vi "grabber.vi"() -> ()   [LabVIEW 2010]
uses:
  scan_specification_tagResonant.ctl
  FPGA_ref.ctl
  <vilib>/Utility/error.llb/DialogType.ctl
  <vilib>/Platform/TimedLoop/XDataNode/XDataNode.xnode
  <vilib>/Platform/TimedLoop/XDataNode/timing_clust.ctl
  <vilib>/Platform/TimedLoop/XDataNode/nitl_modes.ctl
  <vilib>/Platform/TimedLoop/XDataNode/wakeup.ctl
  <vilib>/rvi/interface/nirviReadWriteControl/nirviReadWriteControl.xnode
  <vilib>/rvi/interface/common/niFpgaNodeNameForErrorReporting.ctl
  <vilib>/rvi/errors/niLvFpgaWhatHappensToTopLevelVI.ctl
  tracker status.ctl
  location3D.ctl
  <vilib>/dex/Flush And Wait Empty Condition.ctl
  <vilib>/rvi/interface/nirviMethod/nirviMethod.xnode
  <vilib>/rvi/interface/nirviCloseFPGA/nirviCloseFPGA.xnode
  common/utilities/get_time.vi
  sumLinesIntoVolume.vi
  addLineToVolume.vi
  get write location linear fit.vi
  <vilib>/Utility/error.llb/Error Cluster From Error Code.vi
  <vilib>/rvi/errors/niLvFpgaAdjustHostInterfaceError.vi
  <vilib>/FPGAPlugInAG/Dynamic/niLvFpga_Close_Dynamic.vi
  <vilib>/Platform/TimedLoop/XDataNode/XDNodeRunTimeDep.lvlib
  NiFpgaLv.dll
panel:
  in  "stim delay":i16=-10
  in  "BLEACH!":bool
  in  "Pockels cell bleach":i16=350 min=-750 max=750 step=1
  in  "pockels always on":bool
  in  "ff vel?":bool
  in  "lines per revolution":u16=50
  in  "mark valid location":bool
  in  "reset tracker":bool
  in  "number of spots":u8
  out "filtered spot locations":T1(array[cluster])
  in  "spot location constraints":T2(array[cluster])=[{"spot number"=0, "active"=FALSE, "x max"=0, "x min"=0, "y max"=0, "y min"=0}, {"spot number"=0, "active"=FALSE, "x max"=0, "x min"=0, "y max"=0, "y min"=0}, {"spot number"=0, "active"=FALSE, "x max"=0, "x min"=0, "y max"=0, "y min"=0}, {"spot number"=0, "active"=FALSE, "x max"=0, "x min"=0, "y max"=0, "y min"=0}]
  in  "inter-spot delay":u8
  in  "circles per spot":u16=4
  in  "stim width":u16=24 min=10
  out "stim laser on":bool
  in  "pos to stage lowpass f":dbl=20.0
  in  "measure offset":bool
  in  "Vxy feedback":bool=TRUE
  out "out of range":bool
  in  "auto disable tracking?":bool=TRUE
  in  "out of range (um)":dbl=220.0
  in  "pk-pk tag amplitude (um)":dbl=17.0
  in  "trackingToPiezoScale":fxp<+/-,16,5>=-0.43701171875
  out "current velocity":dbl[](array[numeric])
  out "current position":dbl[](array[numeric])
  in  "z-diff (um^2/ms)":dbl=1.0
  in  "Vz feedback?":bool
  in  "scale factors (um/level)":dbl[](array[numeric])=[0.016, 0.016, 0.00025]
  in  "z-feedback range":i16=5120
  in  "gaussian":bool=TRUE
  in  "x-y phase shift (*2^16/2*pi)":u16=16384
  in  "vmax (um/s)":dbl=10000.0
  in  "Vdiff /(g^2*1ms)":dbl=2e-08
  in  "r sphere/sigma (um)":dbl=3.0
  in  "min photons for update":u32=10
  in  "feedback channel":enum16{"channel 0", "channel 1", "both"}(ring)=enum."both"
  out "idle?":bool
  out "# elements in scan pos queue":i32
  in  "tracking?":bool
  in  "maximum galvo frequency":dbl=3000.0
  in  "scanning mode":enum16{"triangle", "spiral"}(ring)
  in  "LSB has acquire control":bool=TRUE
  in  "AI look-ahead":i16=1300
  in  "delay scan start":u16
  out "Queue Status":T3 {"lines that need sorting" format="%_3p"; "lines that need data" format="%.3p"}
  in  "xyz order":bool
  out "sorter stats":T4
  out "assembler status":T5
  in  "useReadPosition":bool=TRUE
  out "fpga update finished":bool
  out "transfer finished":bool
  out "assembler fin":bool
  out "finished":bool[](array[boolean])
  out "entered":bool[](array[boolean])
  in  "stop":bool
  in  "piezo z feedback":bool=TRUE
  in  "N Image sums":u32=20
  in  "spilt ff/fb":bool
  out "scan specification":T6={"z resolution (pixels)"=100, "iterations per pixel"=28, "iterations per z-scan (=zres*iterperpixel)"=50, "x resolution (pixels)"=100, "y resolution (pixels)"=80, "number of z-lines per volume"=30, "number of repetitions (volumes)"=5, "Pockels cell voltage (bits)"=80, "Vx center (bits)"=0, "Vy center (bits)"=0, "Vx amplitude (bits)"=40, "Vy amplitude (bits)"=0, "lines to delay between scan start and output"=1, "LSB has acquire control"=FALSE, "Pockels cell bleach voltage"=0}
  in  "Pockels cell voltage":i16=85 min=-750 max=750 step=1
  out "number of update commands received":i32
  out "scan spec set":bool
  out "display loop finished":bool
  in  "stop acquisition at FIFO overflow?":bool
  out "scanning? FPGA":bool
  in  "Close front-panel?":bool=TRUE
  out "initialised?":bool
  out "last received command":string
  out "command loop finished":bool
  out "read loop finished":bool
  out "scanning?":bool
  # "Status"
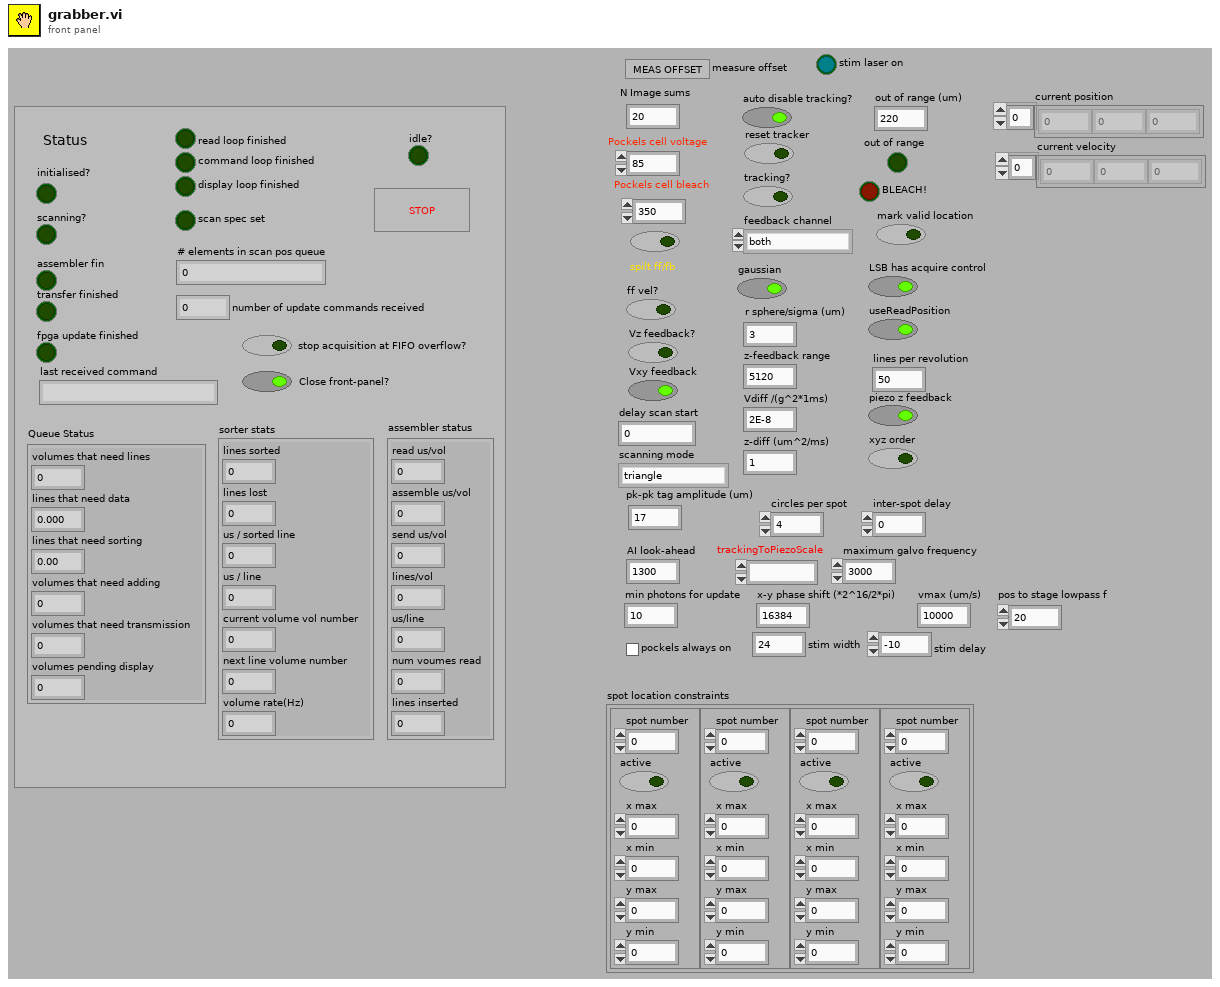
[diagram p1: front panel]
types:
  T1 = cluster{"Filtered x":dbl, "Filtered x":dbl, "Filtered x":dbl}[]
  T2 = cluster{"spot number":i8, "active":bool, "x max":i16, "x min":i16, "y max":i16, "y min":i16}[]
  T3 = cluster{"volumes that need lines":i32, "lines that need data":i32, "lines that need sorting":i32, "volumes that need adding":i32, "volumes that need transmission":i32, "volumes pending display":i32}
  T4 = cluster{"lines sorted":i32, "lines lost":i32, "us / sorted line":dbl, "us / line":dbl, "current volume vol number":u32, "next line volume number":u32, "volume rate(Hz)":dbl}
  T5 = cluster{"read us/vol":dbl, "assemble us/vol":dbl, "send us/vol":dbl, "lines/vol":dbl, "us/line":dbl, "num voumes read":u32, "lines inserted":i32}
  T6 = typedef "scan_specification_tagResonant.ctl" = cluster{"z resolution (pixels)":u16, "iterations per pixel":u16, "iterations per z-scan (=zres*iterperpixel)":u16, "x resolution (pixels)":u16, "y resolution (pixels)":u16, "number of z-lines per volume":u16, "number of repetitions (volumes)":i32, "Pockels cell voltage (bits)":i16, "Vx center (bits)":i16, "Vy center (bits)":i16, "Vx amplitude (bits)":i16, "Vy amplitude (bits)":i16, "lines to delay between scan start and output":u16, "LSB has acquire control":bool, "Pockels cell bleach voltage":i16}
  T7 = typedef "DialogType.ctl" = u16
  T8 = typedef "XDNodeRunTimeDep.lvlib/timing_clust.ctl" = cluster{"Expected End [f-1]":u64, "Actual End [f-1]":u64, "Finished Late? [f-1]":bool, "Expected End [i-1]":u64, "Actual End [i-1]":u64, "Finished Late? [i-1]":bool, "Expected Start [i]":u64, "Actual Start [i]":u64, "Expected Start [f]":u64, "Actual Start [f]":u64, "Source Name":string, "Structure Name":string, "Period":i64, "Deadline":i64, "Offset":i64, "Start":i64, "Priority":i32, "Timeout":i32, "Mode":T9, "Wakeup Reason":T10, "Error":errorcluster, "Source Type":string, "Secondary Source Type":string, "Global End Time":u64, "Global Start Time":u64, "Frame Duration":u64, "Iteration Duration":u64, "Assigned CPU":i32, "I/O Scan Engine Mode":u32}
  T9 = typedef "XDNodeRunTimeDep.lvlib/nitl_modes.ctl" = enum32{"No Change", "Process missed periods, maintain original phase", "Discard missed periods, maintain original phase", "Process missed periods, ignore original phase", "Discard missed periods, ignore original phase"}
  T10 = typedef "XDNodeRunTimeDep.lvlib/wakeup.ctl" = enum32{"Normal", "Aborted", "Asynchronous wakeup", "Timing source error", "Timed loop error", "Timeout"}
  T11 = typedef "internal_queues.ctl" = cluster{"volumeQueue":refnum<queue>, "linesWithoutDataQueue":refnum<queue>, "lineQueue":refnum<queue>, "volumesWithLinesQueue":refnum<queue>, "kalmanQueue":refnum<queue>, "completedVolumeQueue":refnum<queue>, "displayVolumeQueue":refnum<queue>, "scanLocationsQueue":refnum<queue>, "kalmanToDisplayPanel":refnum<queue>, "focalPositionQueue":refnum<queue>, "spotPositionsToImagePanel":refnum<queue>}
  T12 = typedef "network_streaming_queues_cluster.ctl" = cluster{"data writer endpoint":refnum<k21>, "command reader endpoint":refnum<k21>, "settings reader endpoint":refnum<k21>, "z/intensity tuples reader endpoint":refnum<k21>, "extra waitlines reader endpoint":refnum<k21>}
  T13 = typedef "FPGA_ref.ctl" = refnum<k20>
  T14 = cluster{"trackingPanel":refnum<vi>, "imagePanel":refnum<vi>, "fpgaDisplay":refnum<vi>, "stagePanel":refnum<vi>, "filePanel":refnum<vi>, "stimLaserPanel":refnum<vi>}
  T15 = typedef "niFpgaNodeNameForErrorReporting.ctl" = enum16{"Open FPGA VI Reference", "Read/Write Control", "Invoke Method: Abort", "Invoke Method: Acknowledge IRQ", "Invoke Method: Download", "Invoke Method: FIFO.Configure", "Invoke Method: FIFO.Read", "Invoke Method: FIFO.Start", "Invoke Method: FIFO.Stop", "Invoke Method: FIFO.Write", "Invoke Method: Reset", "Invoke Method: Run", "Invoke Method: Wait on IRQ", "Close FPGA VI Reference"}
  T16 = typedef "niLvFpgaWhatHappensToTopLevelVI.ctl" = enum16{"top level VI scripted behind XNode", "top level VI inlined behind XNode"}
  T17 = cluster{"scan specification":T6, "scale factors (um/level)":dbl[], "z-feedback range":i16, "r sphere/sigma (um)":dbl}
  T18 = cluster{"x min":i32, "x max":i32, "y min":i32, "y max":i32, "Active":bool}[]
  T19 = cluster{"x value":i16, "y value":i16, "z value":i16}[]
  T20 = cluster{"z resolution (pixels)":u16, "iterations per pixel":u16, "iterations per z-scan (=zres*iterperpixel)":u16, "x resolution (pixels)":u16, "y resolution (pixels)":u16, "number of z-lines per volume":u16, "number of repetitions (volumes)":i32, "Pockels cell voltage (bits)":i16, "Vx center (bits)":i16, "Vy center (bits)":i16, "Vx amplitude (bits)":i16, "Vy amplitude (bits)":i16, "lines to delay between scan start and output":u16, "LSB has acquire control":bool, "Pockels cell bleach voltage":i16}
  T21 = typedef "tracker status.ctl" = cluster{"scanning":bool, "tracking":bool, "out of range":bool, "stim laser on":bool}
  T22 = cluster{"None":i32, "Volume Start":i32, "Line Start":i32, "COM":i32, "not used":i32}
  T23 = cluster{"command elements pending":u32, "commands read":u32}
  T24 = typedef "location3D.ctl" = cluster{"x (um)":dbl, "y (um)":dbl, "z (um)":dbl, "time (ms)":i64}
  T25 = typedef "kalman_result_scaled.ctl" = cluster{"axis":u8, "pos":dbl, "vel":dbl, "wpe or z_piezo":dbl, "status":u32, "n photon ch 0":u32, "n photon ch 1":u32, "elapsed time":dbl}
  T26 = typedef "polar tracking settings.ctl" = cluster{"scan radius":u16, "2^16/lines per revolution":u16, "gx":fxp<+,16,8>, "rtw":fxp<+,16,26>, "lines per revolution":u8, "vel diff":fxp<+,24,-22>, "Dx - for pos only k-f":fxp<+,32,19>}
  T27 = cluster{"# elements in queue":i32, "# elements in queue":i32, "# elements in queue":i32, "# elements in queue":i32, "# elements in queue":i32, "# elements in queue":i32}
  T28 = typedef "Flush And Wait Empty Condition.ctl" = u8
  T29 = typedef "scan_specification_cluster.ctl" = cluster{"x amplitude":u16, "x resolution (pixels)":u16, "x offset fly-forward (iterations)":u16, "x offset fly-back (iterations)":u16, "y resolution (nr. of lines)":u16, "y step size":u16, "iterations per pixel":u16, "number of frames":i32, "y offset (pixels)":u16, "number of y-brake lines  (before y-fly-back)":u16, "number y-brake lines (after y-fly-back)":u16, "number of y-fly-back steps":u16, "lines per z step":u16, "number of z/intensity tuples":u16, "number of repetitions (volumes or planes)":i32, "z step size derived":u16, "choose the beginning of z scan":bool, "number of frames (settings)":i32, "FPGA trajectory?":bool, "Pockels cell voltage (bits)":i16, "Vy min(bits)":i16, "Vz min(bits)":i16}
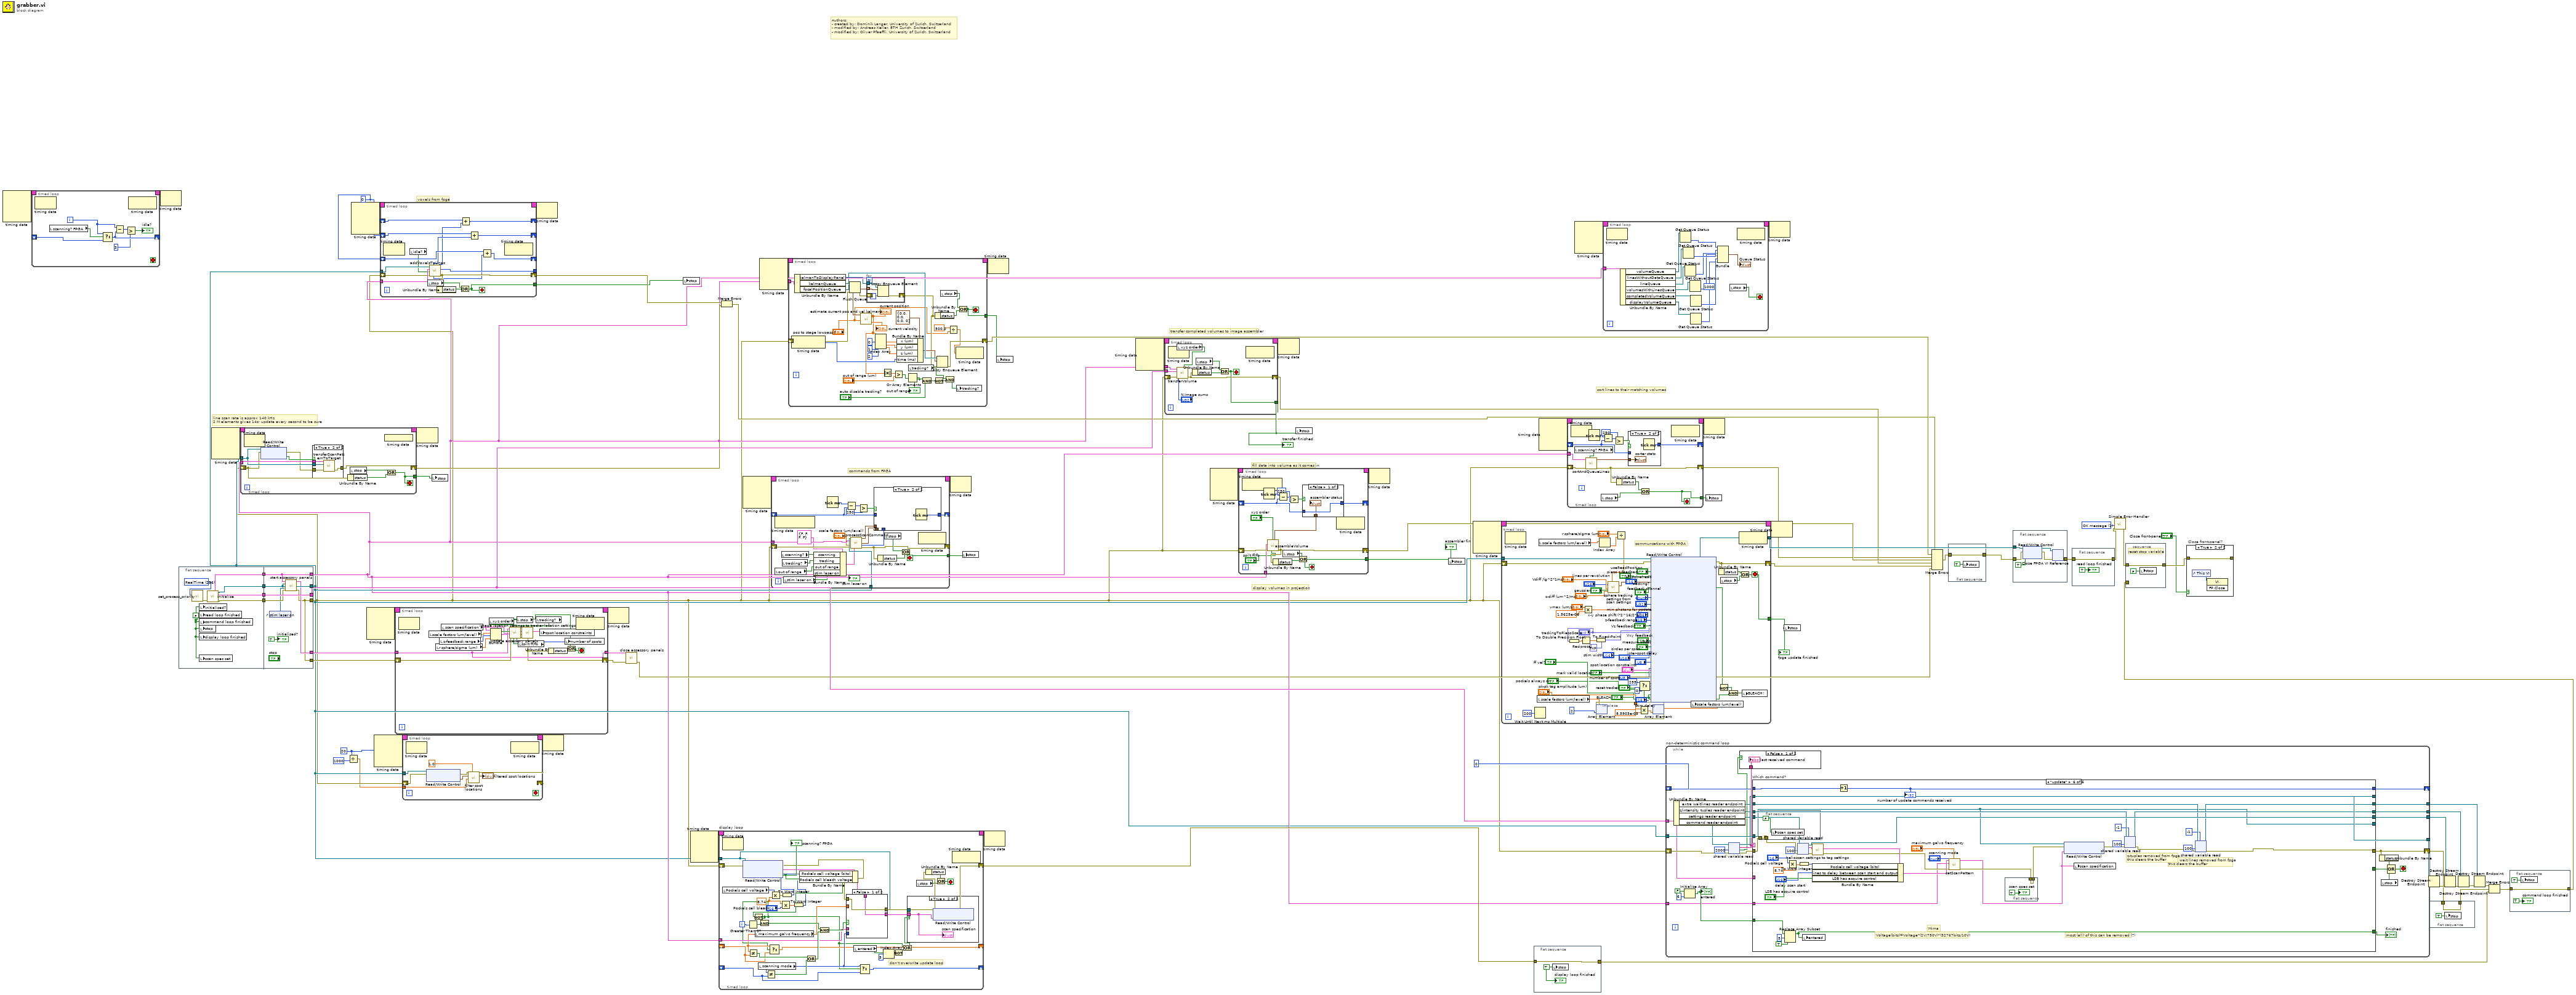
[diagram p0: block diagram]
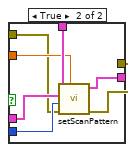
[diagram p3: hidden frame]
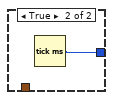
[diagram p6: hidden frame]
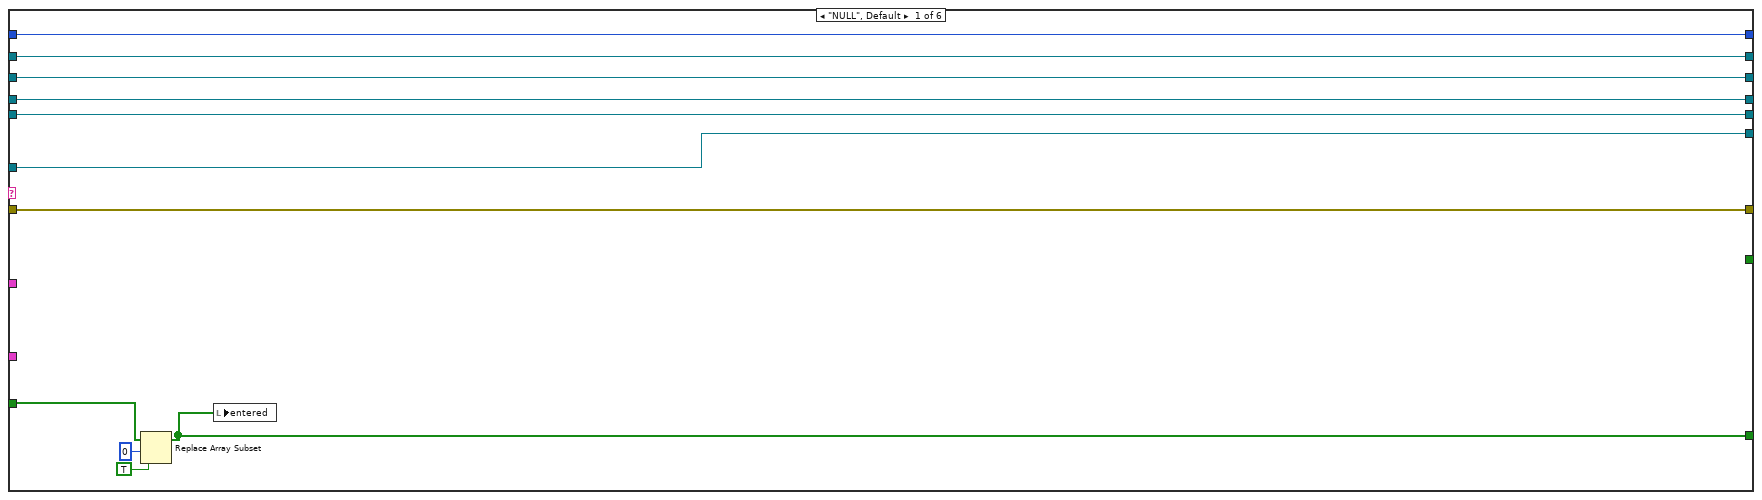
[diagram p10: hidden frame]
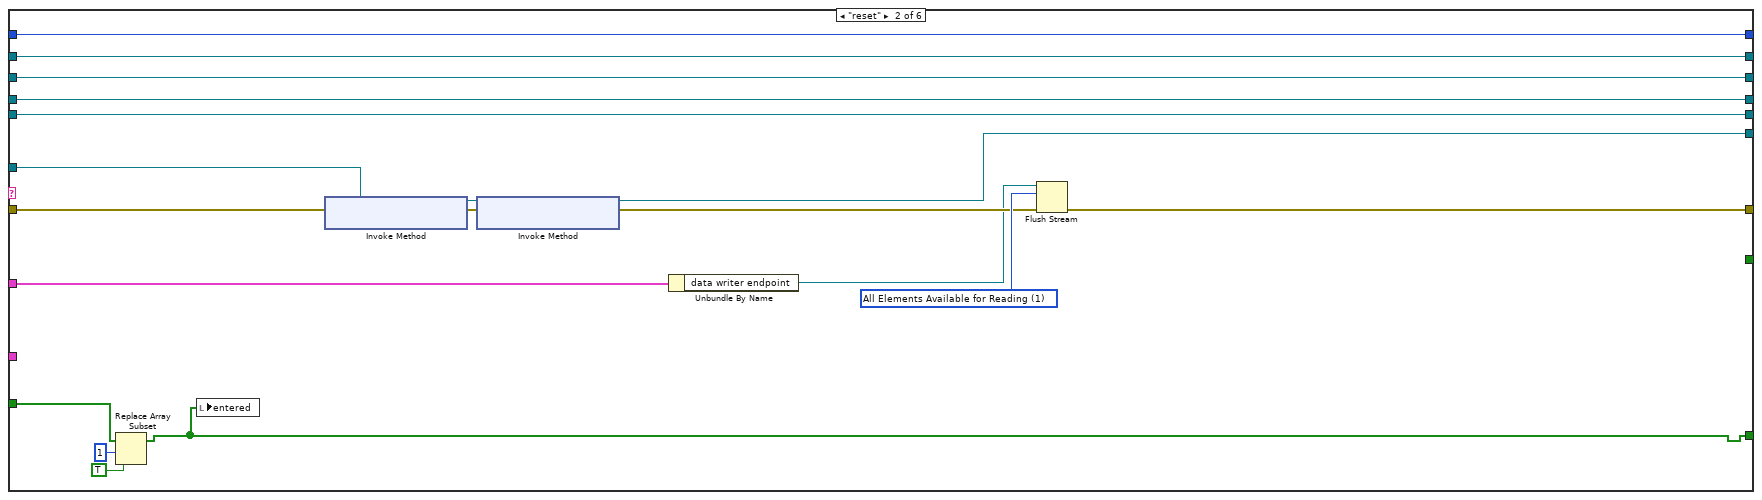
[diagram p11: hidden frame]
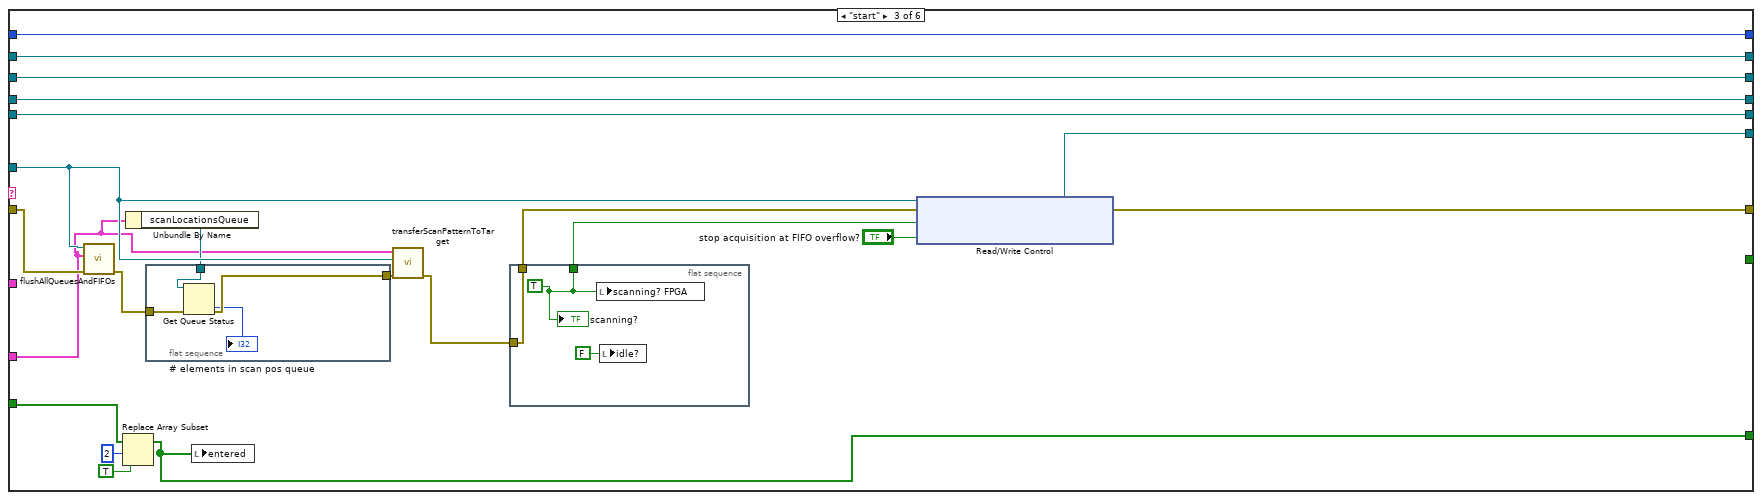
[diagram p12: hidden frame]
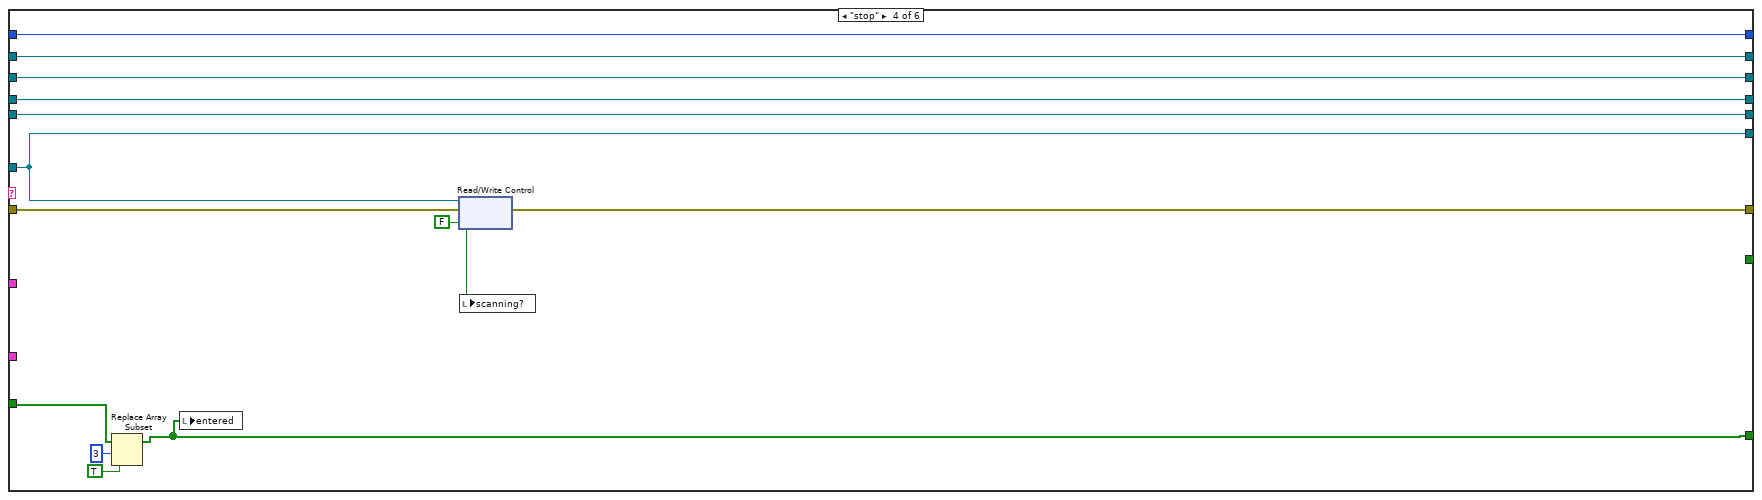
[diagram p13: hidden frame]
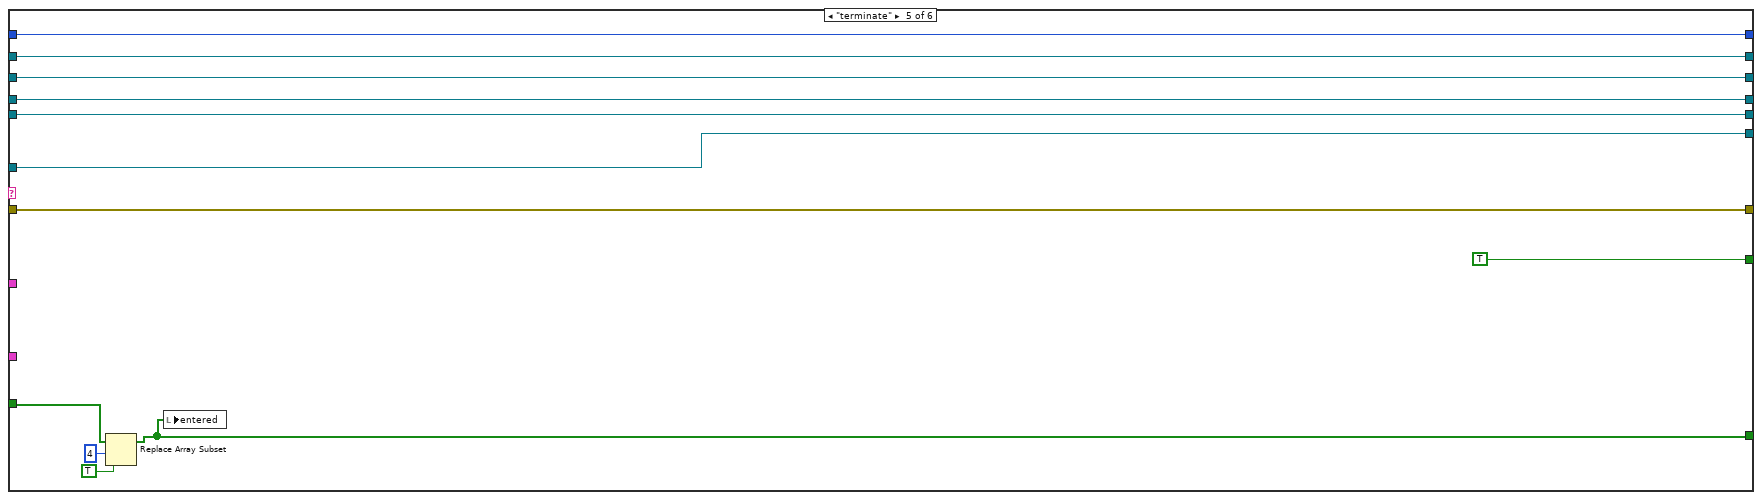
[diagram p14: hidden frame]
diagram:
  w3 = i64 20 ("Period")
  w27 = T7 1 items=["no dialog", "OK message", "continue or stop message", "OK message + warnings", "continue/stop + warnings"] ("type of dialog (OK msg:1)")
  w30 = u32 0
  # "sort lines to their matching volumes"
  # "line scan rate is approx 140 kHz\n2 M elements gives 14s; update every second to be sure"
  # "voxels from fpga"
  # "display volumes in projection"
  # "transfer completed volumes to image assembler"
  # "fill data into volume as it comes in"
  # "commands from FPGA"
  # "Authors: \n- created by: Dominik Langer, University of Zurich, Switzerland\n- modified by: Andreas Keller, ETH Zurich, Switzerland\n- modified by: Oliver Pfaeffli, University of Zurich, Switzerland"
  n1 = node-c288() -> (w23:T8)  [unwired: 4 in]
  n2 = timed-loop {
    timing: w23 -> [_]
    timing-out: [_] -> w22
    shift-right: [w88] -> _
    shift-left: _ -> [w90]
    i -> [w89]
    stop <- _ stop-if-true
    n3 = node-c288() -> ()  [unwired: 1 in, 1 out]
    n4 = local read "scanning? FPGA"() -> (w87:bool)
    n5 = Select(t=w89, s=w87, f=w90) -> (s? t:f=w88:i32)
    n6 = Subtract(x=w89, y=w88) -> (x-y=w86:i32)
    n7 = Greater?(x=w86, y=3) -> (0:→"idle?":bool)
    n8 = node-c288() -> ()  [unwired: 1 in, 1 out]
  }
  n9 = node-c288(w22) -> ()  [unwired: 1 out]
  n10 = flat-sequence {
    tunnel: [w97] -> w80
    tunnel: [w95] -> w79
    tunnel: [w96] -> w77
    tunnel: [w93] -> w61
    tunnel: [w104] -> w5
    tunnel: [w101] -> w4
    tunnel: w80 -> [w103]
    tunnel: w79 -> [w104]
    tunnel: [w106] -> w49
    tunnel: w77 -> [w106]
    tunnel: [w105] -> w31
    tunnel: w61 -> [w105]
    tunnel: [w102] -> w12
    tunnel: [w101] -> w11
    frame #0 {
      w94 = FALSE ("read loop finished")
      w99 = 256 items=["Normal"=32, "Idle"=64, "High"=128, "RealTime"=256, "BelowNormal"=16384, "AboveNormal"=32768] ("PriorityClass")
      n11 = call "set_process_priority.vi"("PriorityClass"=w99) -> ("error out"=w98:errorcluster)  [unwired: 10 in]
      n12 = local write "initialised?"(w94) -> ()
      n13 = local write "read loop finished"(w94) -> ()
      n14 = local write "command loop finished"(w94) -> ()
      n15 = local write "stop"(w94) -> ()
      n16 = local write "display loop finished"(w94) -> ()
      n17 = local write "scan spec set"(w94) -> ()
      n18 = call "initialise.vi"("error in (no error)"=w98) -> ("Queues"=w93:T11, "error out"=w97:errorcluster, "network streaming queues"=w96:T12, "FPGA VI ref"=w95:T13)  [unwired: 5 in, 1 out]
    }
    frame #1 {
      n19 = control-ref of="stim laser on"() -> (w100:refnum<vi>)
      n20 = call "start accessory panels.vi"("error in (no error)"=w103, "stim laser ref"=w100, "FPGA VI ref"=w104, "Queues"=w105) -> ("error out"=w101:errorcluster, "refs"=w102:T14)  [unwired: 6 in]
      "initialised?" <- TRUE ("initialised?")
    }
  }
  n21 = node-c288() -> (w46:T8)  [unwired: 4 in]
  n22 = timed-loop {
    shift-right: [w113] -> w35
    shift-left: w4 -> [w110]
    tunnel: w5 -> [w112]
    timing: w46 -> [_]
    timing-out: [_] -> w45
    tunnel: w31 -> [w114]
    tunnel: [w108] -> w25
    stop <- w108 stop-if-true
    n23 = node-c288() -> ()  [unwired: 1 in, 1 out]
    n24 = xnode "Read/Write Control"("FPGA VI Reference In"=w112, "error in"=w110) -> ("error out"=w109:errorcluster, "scanning?"=w111:bool)  [unwired: 1 out]
    n25 = case shown="True" w111 {
      tunnel: w109 -> [w117 w121]
      tunnel: w114 -> [_ w120]
      tunnel: [w117 w119] -> w113
      tunnel: w112 -> [_ w118]
      frame False {
      }
      frame True {
        n26 = call "transferScanPatternToTarget.vi"("error in (no error)"=w121, "FPGA VI ref"=w118, "Queues"=w120) -> ("error out"=w119:errorcluster)  [unwired: 8 in]
      }
    }
    n27 = Unbundle By Name(w110) -> ("status"=w116:bool)
    n28 = local read "stop"() -> (w115:bool)
    n29 = node-c288() -> ()  [unwired: 1 out]
    n30 = Or(x=w115, y=w116) -> (x .or. y?=w108:bool)
  }
  n31 = Divide(x=w3, y=i64 1000) -> (x/y=w1:dbl)
  n32 = node-c288() -> (w44:T8)  [unwired: 4 in]
  n33 = node-c288() -> (w14:T8)  [unwired: 4 in]
  n34 = node-c288(w3) -> (w7:T8)  [unwired: 3 in]
  n35 = timed-loop {
    timing: w44 -> [_]
    timing-out: [_] -> w43
    tunnel: w5 -> [w184]
    tunnel: w31 -> [w183]
    shift-right: [w178] -> w36
    shift-left: w4 -> [w180]
    tunnel: [w179] -> w26
    shift-right: [w177] -> _
    shift-left: w30 -> [w176]
    shift-right: [w175] -> _
    shift-left: w30 -> [w174]
    tunnel: [w173] -> _
    shift-right: [w169] -> _
    shift-left: w30 -> [w168]
    stop <- w179 stop-if-true
    n36 = node-c288() -> ()  [unwired: 1 in, 1 out]
    n37 = local read "idle?"() -> (w167:bool)
    n38 = local read "stop"() -> (w181:bool)
    n39 = call "addVoxelsToLines.vi"("error in"=w180, "idle?"=w167, "Queues"=w183, "FPGA VI ref"=w184) -> ("error out"=w178:errorcluster, "num elements available"=w173:u32, "num zero volume lines"=w170:u32, "num read"=w171:u32, "lines read"=w172:u32)  [unwired: 1 in, 2 out]
    n40 = Unbundle By Name(w178) -> ("status"=w182:bool)
    n41 = Or(x=w181, y=w182) -> (x .or. y?=w179:bool)
    n42 = Add(x=w168, y=w170) -> (x+y=w169:u32)
    n43 = Add(x=w176, y=w172) -> (x+y=w177:u32)
    n44 = Add(x=w174, y=w171) -> (x+y=w175:u32)
    n45 = node-c288() -> ()  [unwired: 1 in, 1 out]
  }
  n46 = timed-loop {
    timing: w14 -> [_]
    timing-out: [_] -> w13
    tunnel: w12 -> [w197]
    shift-right: [w192] -> w10
    shift-left: w11 -> [w200]
    tunnel: [w197] -> w9
    stop <- w198 stop-if-true
    n47 = node-c288() -> ()  [unwired: 1 in, 1 out]
    n48 = local read "scale factors (um/level)"() -> (w189:dbl[])
    n49 = local read "r sphere/sigma (um)"() -> (w187:dbl)
    n50 = local read "z-feedback range"() -> (w188:i16)
    n51 = local read "scan specification"() -> (w190:T6)
    n52 = local read "xyz order"() -> (w203:bool)
    n53 = Bundle("scan specification"=w190, "scale factors (um/level)"=w189, "z-feedback range"=w188, "r sphere/sigma (um)"=w187) -> (w191:T17)  [unwired: 1 in]
    n54 = local read "stop"() -> (w199:bool)
    n55 = local read "spilt ff/fb"() -> (w202:bool)
    n56 = local read "tracking?"() -> (w196:bool)
    n57 = call "update accessory panels.vi"("tracking"=w196, "spilt ff/fb"=w202, "xyz order"=w203, "error in (no error)"=w200, "scaling info"=w191, "stop"=w199, "refs"=w197) -> ("error out"=w192:errorcluster, "location constraints"=w194:T18, "num spots"=w195:u8)  [unwired: 2 in]
    n58 = call "image location settings to tracker location settings.vi"("scan settings"=w190, "location constraints"=w194) -> ("spot location constraints"=w193:T2)  [unwired: 9 in]
    n59 = local write "spot location constraints"(w193) -> ()
    n60 = Unbundle By Name(w192) -> ("status"=w201:bool)
    n61 = local write "number of spots"(w195) -> ()
    n62 = Or(x=w199, y=w201) -> (x .or. y?=w198:bool)
    n63 = node-c288() -> ()  [unwired: 1 in, 1 out]
  }
  n64 = timed-loop {
    timing: w7 -> [_]
    timing-out: [_] -> w6
    tunnel: w5 -> [w212]
    shift-right: [w209] -> _
    shift-left: w4 -> [w208]
    tunnel: w1 -> [w210]
    stop <- _ stop-if-true
    n65 = node-c288() -> ()  [unwired: 1 in, 1 out]
    n66 = xnode "Read/Write Control"("FPGA VI Reference In"=w212, "error in"=w208) -> ("error out"=w209:errorcluster, "Spot locations"=w211:T19)  [unwired: 1 out]
    n67 = call "filter spot locations.vi"("high cutoff freq: fh"=1.0, "sampling freq: fs"=w210, "Spot locations"=w211) -> ("filtered spot locations"=→"filtered spot locations":T1)  [unwired: 8 in]
    n68 = node-c288() -> ()  [unwired: 1 in, 1 out]
  }
  n69 = node-c288(w45) -> ()  [unwired: 1 out]
  n70 = local write "stop"(w25) -> ()
  n71 = node-c288(w43) -> ()  [unwired: 1 out]
  n72 = node-c288(w6) -> ()  [unwired: 1 out]
  n73 = node-c288(w13) -> ()  [unwired: 1 out]
  n74 = call "close accessory panels.vi"("error in (no error)"=w10, "refs"=w9) -> ("error out"=w8:errorcluster)  [unwired: 9 in]
  n75 = local write "stop"(w26) -> ()
  n76 = node-c288() -> (w17:T8)  [unwired: 4 in]
  n77 = timed-loop "display loop" {
    tunnel: w5 -> [w276]
    shift-right: [w288] -> w70
    shift-left: w4 -> [w302]
    shift-right: [w282] -> _
    shift-left: _ -> [w284]
    shift-right: [w285] -> _
    shift-left: _ -> [w287]
    tunnel: w31 -> [w290]
    timing: w17 -> [_]
    timing-out: [_] -> w16
    i -> [w298]
    stop <- w299 stop-if-true
    w268 = 8.74 ("x")
    # "don't overwrite update loop"
    n78 = node-c288() -> ()  [unwired: 1 in, 1 out]
    n79 = local read "Pockels cell voltage"() -> (w281:i16)
    n80 = xnode "Read/Write Control"("FPGA VI Reference In"=w276, "error in"=w302) -> ("error out"=w289:errorcluster, "scan specification"=w278:T20, "scanning?"=w296:bool)  [unwired: 1 out]
    "scanning? FPGA" <- w296
    n81 = Greater Than 0?(x=w298) -> (x > 0?=w297:bool)
    n82 = Not(x=w296) -> (.not. x?=w270:bool)
    n83 = local read "maximum galvo frequency"() -> (w283:dbl)
    n84 = Not Equal?(x=w283, y=w284) -> (x != y?=w294:bool)
    n85 = local read "scanning mode"() -> (w286:enum16{"triangle", "spiral"})
    n86 = And(x=w270, y=w297) -> (x .and. y?=w292:bool)
    n87 = Not Equal?(x=w286, y=w287) -> (x != y?=w295:bool)
    n88 = Select(t=w283, s=w270, f=w284) -> (s? t:f=w282:dbl)
    n89 = Multiply(x=w281, y=w268) -> (x*y=w280:dbl)
    n90 = Multiply(x=w268, y="Pockels cell bleach") -> (x*y=w266:dbl)
    n91 = To Word Integer(number=w280) -> (16bit integer=w279:i16)
    n92 = To Word Integer(number=w266) -> (16bit integer=w265:i16)
    n93 = Bundle By Name(cluster=w278, "Pockels cell voltage (bits)"=w279, "Pockels cell bleach voltage"=w265) -> (w277:T20)
    n94 = Or(x=w294, y=w295) -> (x .or. y?=w293:bool)
    n95 = And(x=w292, y=w293) -> (x .and. y?=w291:bool)
    n96 = case shown="False" w291 {
      tunnel: w277 -> [w351 w359]
      tunnel: w283 -> [_ w358]
      tunnel: w286 -> [_ w357]
      tunnel: w290 -> [_ w356]
      tunnel: [w352 w354] -> w288
      tunnel: w289 -> [w352 w355]
      tunnel: [w351 w353] -> w275
      frame False {
      }
      frame True {
        n97 = call "setScanPattern.vi"("maximum frequency"=w358, "error in (no error)"=w355, "scanning mode"=w357, "Queues"=w356, "scan specification - tag resonant"=w359) -> ("error out"=w354:errorcluster, "scan specification out"=w353:T6)  [unwired: 5 in]
      }
    }
    n98 = local read "entered"() -> (w274:bool[])
    n99 = Select(t=w286, s=w270, f=w287) -> (s? t:f=w285:enum16{"triangle", "spiral"})
    n100 = Index Array(array=w274, index=5) -> (element=w273:bool)
    n101 = Not(x=w273) -> (.not. x?=w271:bool)
    n102 = Or(x=w270, y=w271) -> (x .or. y?=w269:bool)
    n103 = case shown="True" w269 {
      tunnel: w276 -> [_ w304]
      tunnel: w275 -> [_ w303]
      frame False {
      }
      frame True {
        n104 = xnode "Read/Write Control"("FPGA VI Reference In"=w304, "scan specification"=w303) -> ()  [unwired: 1 in, 2 out]
        "scan specification" <- w303
      }
    }
    n105 = local read "stop"() -> (w300:bool)
    n106 = Unbundle By Name(w288) -> ("status"=w301:bool)
    n107 = Or(x=w301, y=w300) -> (x .or. y?=w299:bool)
    n108 = node-c288() -> ()  [unwired: 1 in, 1 out]
  }
  n109 = Merge Errors(w36, w35) -> (w34:errorcluster)
  n110 = node-c288() -> (w60:T8)  [unwired: 4 in]
  n111 = node-c288() -> (w21:T8)  [unwired: 4 in]
  n112 = timed-loop {
    tunnel: w5 -> [w458]
    shift-right: [w454] -> _
    shift-left: w4 -> [w455]
    timing: w60 -> [_]
    timing-out: [_] -> w59
    tunnel: w31 -> [w452]
    tunnel: [w453] -> w55
    shift-right: [w449] -> _
    shift-left: _ -> [w447]
    stop <- w453 stop-if-true
    n113 = node-c288() -> ()  [unwired: 1 in, 1 out]
    n114 = local read "out of range"() -> (w439:bool)
    n115 = local read "scanning?"() -> (w441:bool)
    n116 = local read "tracking?"() -> (w440:bool)
    n117 = local read "stim laser on"() -> (w438:bool)
    n118 = Bundle By Name(cluster=T21 {"scanning"=FALSE, "tracking"=FALSE, "out of range"=FALSE, "stim laser on"=FALSE} ("tracker status"), "scanning"=w441, "tracking"=w440, "out of range"=w439, "stim laser on"=w438) -> (w437:T21)
    n119 = Tick Count (ms)() -> (millisecond timer value=w448:u32)
    n120 = Subtract(x=w448, y=w447) -> (x-y=w446:u32)
    n121 = call "processScanCommand.vi"("FPGA VI Reference In"=w458, "Queues"=w452, "scale factors (um/level)"="scale factors (um/level)", "error in (no error)"=w455, "tracker status"=w437) -> ("num calls"=w451:T22, "command queue status"=w450:T23, "num kalmans per axis"=w436:u32[], "error out"=w454:errorcluster)  [unwired: 3 in, 4 out]
    n122 = Greater?(x=w446, y=u32 250) -> (0:w444:bool)
    n123 = case shown="True" w444 {
      tunnel: w451 -> [_ _]
      tunnel: w450 -> [_ _]
      tunnel: [w459 w460] -> w449
      tunnel: w447 -> [w459 _]
      tunnel: w436 -> [_ _]
      frame False {
      }
      frame True {
        n124 = Tick Count (ms)() -> (millisecond timer value=w460:u32)
      }
    }
    n125 = Unbundle By Name(w454) -> ("status"=w457:bool)
    n126 = local read "stop"() -> (w456:bool)
    n127 = Or(x=w456, y=w457) -> (x .or. y?=w453:bool)
    n128 = node-c288() -> ()  [unwired: 1 in, 1 out]
  }
  n129 = timed-loop {
    tunnel: w31 -> [w497]
    shift-right: [w476] -> w37
    shift-left: w4 -> [w495]
    timing: w21 -> [_]
    timing-out: [_] -> w20
    tunnel: [w488] -> w15
    stop <- w488 stop-if-true
    n130 = node-c288() -> (w480:i64)  [unwired: 1 in]
    n131 = Unbundle By Name(w497) -> ("kalmanToDisplayPanel"=w493:refnum<queue>, "kalmanQueue"=w496:refnum<queue>, "focalPositionQueue"=w479:refnum<queue>)
    n132 = Flush Queue(queue=w496, error in (no error)=w495) -> (remaining elements=w492:T25[], error out=w494:errorcluster)  [unwired: 1 out]
    n133 = call "estimate current pos and vel kalman.vi"("feedback lowpass f"="pos to stage lowpass f", "kalman updates"=w492) -> ("current velocity"=→"current velocity":dbl[], "current position"=w475:dbl[])  [unwired: 8 in]
    "current position" <- w475
    n134 = for {
      tunnel: w492 -> [w500] mode=indexing
      tunnel: w493 -> [w501]
      shift-right: [w498] -> w477
      shift-left: w494 -> [w499]
      n135 = Lossy Enqueue Element(queue=w501, element=w500, error in (no error)=w499) -> (error out=w498:errorcluster)  [unwired: 3 out]
    }
    n136 = Index Array(array=w475, index #1=0 ("index"), index #2=1 ("index"), index #3=2 ("index")) -> (element #1=w483:dbl, element #2=w482:dbl, element #3=w481:dbl)
    n137 = Absolute Value(x=w475) -> (abs(x)=w474:dbl[])
    n138 = Greater?(x=w474, y="out of range (um)") -> (0:w472:bool[])
    n139 = Bundle By Name(cluster=T24 {"x (um)"=0.0, "y (um)"=0.0, "z (um)"=0.0, "time (ms)"=0} ("location"), "x (um)"=w483, "y (um)"=w482, "z (um)"=w481, "time (ms)"=w480) -> (w478:T24)
    n140 = Or Array Elements(Boolean array=w472) -> (logical OR=w471:bool)
    "out of range" <- w471
    n141 = local read "tracking?"() -> (w467:bool)
    n142 = And(x=w471, y="auto disable tracking?") -> (x .and. y?=w469:bool)
    n143 = Not(x=w469) -> (.not. x?=w468:bool)
    n144 = Unbundle By Name(w477) -> ("status"=w490:bool)
    n145 = Lossy Enqueue Element(queue=w479, element=w478, error in (no error)=w477) -> (error out=w476:errorcluster)  [unwired: 3 out]
    n146 = local read "stop"() -> (w489:bool)
    n147 = And(x=w467, y=w468) -> (x .and. y?=w466:bool)
    n148 = Divide(x=500.0, y="pos to stage lowpass f") -> (x/y=w463:dbl)
    n149 = node-c288(w463) -> ()  [unwired: 1 out]
    n150 = local write "tracking?"(w466) -> ()
    n151 = Or(x=w489, y=w490) -> (x .or. y?=w488:bool)
  }
  n152 = node-c288(w59) -> ()  [unwired: 1 out]
  n153 = local write "stop"(w55) -> ()
  n154 = node-c288(w16) -> ()  [unwired: 1 out]
  n155 = node-c288(w20) -> ()  [unwired: 1 out]
  n156 = local write "stop"(w15) -> ()
  n157 = node-c288() -> (w40:T8)  [unwired: 4 in]
  n158 = timed-loop {
    tunnel: w31 -> [w508]
    shift-right: [w510] -> w48
    shift-left: w4 -> [w515]
    tunnel: [w512] -> w47
    tunnel: w49 -> [w509]
    timing: w40 -> [_]
    timing-out: [_] -> w39
    stop <- w512 stop-if-true
    n159 = node-c288() -> ()  [unwired: 1 in, 1 out]
    n160 = local read "xyz order"() -> (w507:bool)
    n161 = call "transferVolume.vi"("xyz order"=w507, "error in (no error)"=w515, "num vol to sum"="N Image sums", "network streaming queues"=w509, "Queues"=w508) -> ("error out"=w510:errorcluster)  [unwired: 1 in, 5 out]
    n162 = Unbundle By Name(w510) -> ("status"=w514:bool)
    n163 = local read "stop"() -> (w513:bool)
    n164 = Or(x=w513, y=w514) -> (x .or. y?=w512:bool)
    n165 = node-c288() -> ()  [unwired: 1 in, 1 out]
  }
  "transfer finished" <- w47
  n166 = node-c288() -> (w58:T8)  [unwired: 4 in]
  n167 = timed-loop {
    timing: w58 -> [_]
    timing-out: [_] -> w57
    tunnel: w31 -> [w527]
    shift-right: [w528] -> w53
    shift-left: w4 -> [w532]
    tunnel: [w529] -> w56
    shift-right: [w526] -> _
    shift-left: _ -> [w521]
    stop <- w529 stop-if-true
    n168 = node-c288() -> ()  [unwired: 1 in, 1 out]
    n169 = Tick Count (ms)() -> (millisecond timer value=w525:u32)
    n170 = call "assembleVolume.vi"("calc ff/fb"="spilt ff/fb", "error in (no error)"=w532, "xyz order"="xyz order", "Queues"=w527) -> ("error out"=w528:errorcluster, "status"=w520:T5)  [unwired: 5 in, 1 out]
    n171 = Unbundle By Name(w528) -> ("status"=w531:bool)
    n172 = Subtract(x=w525, y=w521) -> (x-y=w524:u32)
    n173 = local read "stop"() -> (w530:bool)
    n174 = Greater?(x=w524, y=u32 250) -> (0:w522:bool)
    n175 = Or(x=w530, y=w531) -> (x .or. y?=w529:bool)
    n176 = case shown="False" w522 {
      tunnel: [w534 w535] -> w526
      tunnel: w521 -> [w534 _]
      tunnel: w520 -> [w533 _]
      frame False {
        "assembler status" <- w533
      }
      frame True {
        n177 = Tick Count (ms)() -> (millisecond timer value=w535:u32)
      }
    }
    n178 = node-c288() -> ()  [unwired: 1 in, 1 out]
  }
  "assembler fin" <- w56
  n179 = node-c288(w39) -> ()  [unwired: 1 out]
  n180 = local write "stop"(w47) -> ()
  n181 = node-c288(w57) -> ()  [unwired: 1 out]
  n182 = local write "stop"(w56) -> ()
  n183 = node-c288() -> (w19:T8)  [unwired: 4 in]
  n184 = timed-loop {
    tunnel: w5 -> [w592]
    shift-right: [w555] -> w54
    shift-left: w4 -> [w591]
    tunnel: [w587] -> w51
    tunnel: [w586] -> w50
    timing: w19 -> [_]
    timing-out: [_] -> w18
    stop <- w586 stop-if-true
    # "communcations with FPGA"
    n185 = node-c288() -> ()  [unwired: 1 in, 1 out]
    n186 = Wait Until Next ms Multiple(millisecond multiple=u32 200) -> ()  [unwired: 1 out]
    n187 = local read "scale factors (um/level)"() -> (w566:dbl[])
    n188 = local read "scale factors (um/level)"() -> (w559:dbl[])
    n189 = To Double Precision Float(number="trackingToPiezoScale") -> (double precision float=w570:dbl)
    n190 = Reciprocal(x=w570) -> (1/x=w569:dbl)
    n191 = Multiply(x="vmax (um/s)", y=1.5625e-06) -> (x*y=w577:dbl)
    n192 = To Fixed-Point(fixed-point type=fxp<+/-,16,2> 0.0 ("piezoToTrackingScale"), number=w569) -> (fixed-point=w568:fxp<+/-,16,2>)
    n193 = in-place {
      in-place-border: "pk-pk tag amplitude (um)" -> [w596]
      n194 = in-place-array #1(w566, 2) -> ()  [unwired: 1 out]
      n195 = Multiply(x=w596, y=8.5903e-05) -> (x*y=w594:dbl)
      n196 = in-place-array #1(w594) -> (w565:dbl[])  [unwired: 1 out]
    }
    n197 = Index Array(array=w559) -> (element=w558:dbl)  [unwired: 1 in]
    n198 = Divide(x="r sphere/sigma (um)", y=w558) -> (x/y=w561:dbl)
    n199 = call "sphere tracking settings from scan settings.vi"("gaussian"="gaussian", "sphere radius/sigma"=w561, "z-diff (um^2/ms)"="z-diff (um^2/ms)", "Vdiff /(g^2*1ms)"="Vdiff /(g^2*1ms)", "lines per revolution"="lines per revolution") -> ("tracking settings out"=w581:T26)  [unwired: 6 in]
    n200 = Select(t=u8 255, s="reset tracker", f=u8 0) -> (s? t:f=w549:u8)
    n201 = xnode "Read/Write Control"("FPGA VI Reference In"=w592, "error in"=w591, "piezo z feedback"="piezo z feedback", "useReadPosition"="useReadPosition", "AI look-ahead"="AI look-ahead", "tracking settings"=w581, "tracking?"="tracking?", "feedback channel"="feedback channel", "min photons for update"="min photons for update", "vmax"=w577, "x-y phase shift (*2^16/2*pi)"="x-y phase shift (*2^16/2*pi)", "half valid z-range (ncycles * 64)"="z-feedback range", "Vz feedback?"="Vz feedback?", "trackingToPiezoScale"="trackingToPiezoScale", "piezoToTrackingScale"=w568, "Vxy feedback"="Vxy feedback", "measure offset"="measure offset", "stim buffer counts"="stim width", "circles per spot"="circles per spot", "inter-spot delay"="inter-spot delay", "spot location constraints"="spot location constraints", "number of spots"="number of spots", "reset flags"=w549, "mark valid location"="mark valid location", "ff vel?"="ff vel?", "pockels always on"="pockels always on", "bleach mode"="BLEACH!", "stim delay"="stim delay") -> ("FPGA VI Reference Out"=w587:T13, "error out"=w555:errorcluster)
    n202 = local write "scale factors (um/level)"(w565) -> ()
    n203 = Not(x="tracking?") -> (.not. x?=w540:bool)
    n204 = Unbundle By Name(w555) -> ("status"=w589:bool)
    n205 = local read "stop"() -> (w588:bool)
    n206 = And(x=w540, y="BLEACH!") -> (x .and. y?=w542:bool)
    n207 = node-c288() -> ()  [unwired: 1 in, 1 out]
    n208 = Or(x=w589, y=w588) -> (x .or. y?=w586:bool)
    n209 = local write "BLEACH!"(w542) -> ()
  }
  "fpga update finished" <- w50
  n210 = flat-sequence {
    tunnel: w70 -> [w1209]
    tunnel: [w1209] -> w69
    frame #0 {
      w1208 = TRUE ("stop")
      n211 = local write "stop"(w1208) -> ()
      "display loop finished" <- w1208
    }
  }
  n212 = node-c288() -> (w42:T8)  [unwired: 4 in]
  n213 = timed-loop {
    tunnel: w31 -> [w1222]
    shift-right: [w1221] -> w38
    shift-left: w4 -> [w1223]
    timing: w42 -> [_]
    timing-out: [_] -> w41
    shift-right: [w1216] -> _
    shift-left: _ -> [w1211]
    tunnel: [w1210] -> w24
    stop <- w1210 stop-if-true
    n214 = node-c288() -> ()  [unwired: 1 in, 1 out]
    n215 = local read "scanning? FPGA"() -> (w1217:bool)
    n216 = call "sortAndQueueLines.vi"("scanning?"=w1217, "error in (no error)"=w1223, "Queues"=w1222) -> ("error out"=w1221:errorcluster, "stats"=w1218:T4)  [unwired: 5 in, 2 out]
    n217 = Tick Count (ms)() -> (millisecond timer value=w1215:u32)
    n218 = local read "stop"() -> (w1219:bool)
    n219 = Subtract(x=w1215, y=w1211) -> (x-y=w1214:u32)
    n220 = Greater?(x=w1214, y=u32 250) -> (0:w1212:bool)
    n221 = Unbundle By Name(w1221) -> ("status"=w1220:bool)
    n222 = case shown="True" w1212 {
      tunnel: w1218 -> [_ w1226]
      tunnel: [w1224 w1225] -> w1216
      tunnel: w1211 -> [w1224 _]
      frame False {
      }
      frame True {
        n223 = Tick Count (ms)() -> (millisecond timer value=w1225:u32)
        "sorter stats" <- w1226
      }
    }
    n224 = Or(x=w1220, y=w1219) -> (x .or. y?=w1210:bool)
    n225 = node-c288() -> ()  [unwired: 1 in, 1 out]
  }
  n226 = node-c288() -> (w33:T8)  [unwired: 4 in]
  n227 = timed-loop {
    timing: w33 -> [_]
    timing-out: [_] -> w32
    tunnel: w31 -> [w1243]
    stop <- w1233 stop-if-true
    (unwired) 1000 ("y")
    n228 = node-c288() -> ()  [unwired: 1 in, 1 out]
    n229 = Unbundle By Name(w1243) -> ("volumeQueue"=w1242:refnum<queue>, "linesWithoutDataQueue"=w1241:refnum<queue>, "lineQueue"=w1240:refnum<queue>, "volumesWithLinesQueue"=w1239:refnum<queue>, "completedVolumeQueue"=w1238:refnum<queue>, "displayVolumeQueue"=w1237:refnum<queue>)
    n230 = Get Queue Status(queue=w1242) -> (# elements in queue=w1236:i32)  [unwired: 2 in, 7 out]
    n231 = Get Queue Status(queue=w1241) -> (# elements in queue=w1235:i32)  [unwired: 2 in, 7 out]
    n232 = Get Queue Status(queue=w1240) -> (# elements in queue=w1232:i32)  [unwired: 2 in, 7 out]
    n233 = Get Queue Status(queue=w1239) -> (# elements in queue=w1231:i32)  [unwired: 2 in, 7 out]
    n234 = Get Queue Status(queue=w1237) -> (# elements in queue=w1229:i32)  [unwired: 2 in, 7 out]
    n235 = Get Queue Status(queue=w1238) -> (# elements in queue=w1230:i32)  [unwired: 2 in, 7 out]
    n236 = Bundle("# elements in queue"=w1236, "# elements in queue"=w1235, "# elements in queue"=w1232, "# elements in queue"=w1231, "# elements in queue"=w1230, "# elements in queue"=w1229) -> (→"Queue Status":T27)  [unwired: 1 in]
    n237 = local read "stop"() -> (w1233:bool)
    n238 = node-c288() -> ()  [unwired: 1 in, 1 out]
  }
  n239 = while "non-deterministic command loop" {
    shift-right: [w1260] -> w68
    shift-left: w4 -> [w1273]
    tunnel: w5 -> [w1272]
    tunnel: [w1268] -> w83
    tunnel: w49 -> [w1266]
    tunnel: [w1264] -> w74
    tunnel: [w1262] -> w72
    tunnel: [w1255] -> w64
    shift-right: [w1253] -> _
    shift-left: 0 -> [w1254]
    tunnel: w31 -> [w1247]
    stop <- w1258 stop-if-true
    n240 = Unbundle By Name(w1266) -> ("extra waitlines reader endpoint"=w1256:refnum<k21>, "z/intensity tuples reader endpoint"=w1263:refnum<k21>, "settings reader endpoint"=w1265:refnum<k21>, "command reader endpoint"=w1267:refnum<k21>)
    n241 = Initialize Array(FALSE, 6 ("dimension size")) -> (w1249:bool[])
    "entered" <- w1249
    n242 = shared-variable-read(w1267, w1273, 2000 ("timeout in ms (-1)")) -> (w1269:refnum<k21>, w1271:errorcluster, w1246:bool, w1270:string)
    n243 = case shown="False" w1246 {
      tunnel: w1270 -> [w1274 _]
      frame False {
        "last received command" <- w1274
      }
      frame True {
      }
    }
    n244 = case "Which command?" shown="\"update\"" w1270 {
      tunnel: w1272 -> [w1283 w1302 w1356 w1449 w1500 w1504]
      tunnel: w1271 -> [w1285 w1304 w1357 w1448 w1499 w1530]
      tunnel: [w1285 w1296 w1369 w1446 w1499 w1503] -> w1260
      tunnel: w1269 -> [w1284 w1303 w1368 w1450 w1501 w1540]
      tunnel: [w1284 w1303 w1368 w1450 w1501 w1540] -> w1268
      tunnel: [w1283 w1301 w1367 w1449 w1500 w1504] -> _
      tunnel: w1266 -> [_ w1295 _ _ _ _]
      tunnel: w1265 -> [w1282 w1293 w1366 w1445 w1498 w1539]
      tunnel: [w1282 w1293 w1366 w1445 w1498 w1538] -> w1264
      tunnel: w1263 -> [w1281 w1292 w1365 w1444 w1497 w1537]
      tunnel: [w1281 w1292 w1365 w1444 w1497 w1536] -> w1262
      tunnel: [_ _ _ _ TRUE _] -> w1261
      tunnel: w1256 -> [w1280 w1291 w1364 w1443 w1495 w1534]
      tunnel: [w1280 w1291 w1364 w1443 w1495 w1533] -> w1255
      tunnel: w1254 -> [w1279 w1290 w1362 w1442 w1494 w1528]
      tunnel: [w1279 w1290 w1362 w1442 w1494 w1527] -> w1253
      tunnel: [w1275 w1286 w1358 w1438 w1490 w1517] -> w1250
      tunnel: w1249 -> [w1276 w1287 w1359 w1439 w1491 w1515]
      tunnel: w1247 -> [_ _ w1352 _ _ w1507]
      frame "NULL", Default {
        n245 = Replace Array Subset(array=w1276, new element=TRUE ("new element/subarray"), index=0) -> (w1275:bool[])
        n246 = local write "entered"(w1275) -> ()
      }
      frame "reset" {
        w1298 = T28 1 items=["All Elements Read From Stream", "All Elements Available for Reading"] ("wait condition")
        n247 = Replace Array Subset(array=w1287, new element=TRUE ("new element/subarray"), index=1) -> (w1286:bool[])
        n248 = local write "entered"(w1286) -> ()
        n249 = xnode "Invoke Method"("FPGA VI Reference In"=w1302, "error in"=w1304) -> ("FPGA VI Reference Out"=w1299:T13, "error out"=w1300:errorcluster)
        n250 = xnode "Invoke Method"("FPGA VI Reference In"=w1299, "error in"=w1300) -> ("FPGA VI Reference Out"=w1301:T13, "error out"=w1297:errorcluster)
        n251 = Unbundle By Name(w1295) -> ("data writer endpoint"=w1294:refnum<k21>)
        n252 = Flush Stream(8:w1297, 10:w1298, 11:w1294) -> (0:w1296:errorcluster)  [unwired: 1 in, 2 out]
      }
      frame "start" {
        n253 = call "flushAllQueuesAndFIFOs.vi"("error in (no error)"=w1357, "Queues"=w1352, "FPGA VI ref"=w1356) -> ("error out"=w1355:errorcluster)  [unwired: 8 in]
        n254 = Replace Array Subset(array=w1359, new element=TRUE ("new element/subarray"), index=2) -> (w1358:bool[])
        n255 = Unbundle By Name(w1352) -> ("scanLocationsQueue"=w1353:refnum<queue>)
        n256 = flat-sequence {
          tunnel: w1355 -> [w1376]
          tunnel: [w1375] -> w1354
          tunnel: w1353 -> [w1374]
          frame #0 {
            n257 = Get Queue Status(queue=w1374, error in (no error)=w1376) -> (error out=w1375:errorcluster, # elements in queue=→"# elements in scan pos queue":i32)  [unwired: 1 in, 6 out]
          }
        }
        n258 = local write "entered"(w1358) -> ()
        n259 = call "transferScanPatternToTarget.vi"("error in (no error)"=w1354, "FPGA VI ref"=w1356, "Queues"=w1352) -> ("error out"=w1350:errorcluster)  [unwired: 8 in]
        n260 = flat-sequence {
          tunnel: [w1371] -> w1351
          tunnel: w1350 -> [w1370]
          tunnel: [w1370] -> w1349
          frame #0 {
            w1371 = TRUE ("scan")
            n261 = local write "scanning? FPGA"(w1371) -> ()
            n262 = local write "idle?"(FALSE ("idle?")) -> ()
            "scanning?" <- w1371
          }
        }
        n263 = xnode "Read/Write Control"("FPGA VI Reference In"=w1356, "error in"=w1349, "scan"=w1351, "stop acquisition at FIFO overflow?"="stop acquisition at FIFO overflow?") -> ("FPGA VI Reference Out"=w1367:T13, "error out"=w1369:errorcluster)
      }
      frame "stop" {
        w1447 = FALSE ("scan")
        n264 = Replace Array Subset(array=w1439, new element=TRUE ("new element/subarray"), index=3) -> (w1438:bool[])
        n265 = local write "entered"(w1438) -> ()
        n266 = xnode "Read/Write Control"("FPGA VI Reference In"=w1449, "error in"=w1448, "scan"=w1447) -> ("error out"=w1446:errorcluster)  [unwired: 1 out]
        n267 = local write "scanning?"(w1447) -> ()
      }
      frame "terminate" {
        n268 = Replace Array Subset(array=w1491, new element=TRUE ("new element/subarray"), index=4) -> (w1490:bool[])
        n269 = local write "entered"(w1490) -> ()
      }
      frame "update" {
        # "most (all) of this can be removed (?)"
        # "extra wait lines removed from fpga\nthis clears the buffer"
        # "z-tuples removed from fpga\nthis clears the buffer"
        # "Mirna"
        # "Voltage(bits)=Voltage*(2V/750V)*(32767bits/10V)"
        n270 = flat-sequence {
          tunnel: w1530 -> [w1541]
          tunnel: [w1541] -> w1529
          frame #0 {
            n271 = local write "scan spec set"(FALSE ("extra wait lines set")) -> ()
          }
        }
        n272 = Replace Array Subset(array=w1515, new element=TRUE ("new element/subarray"), index=5) -> (w1517:bool[])
        n273 = Multiply(x="Pockels cell voltage", y=8.74 ("x")) -> (x*y=w1524:dbl)
        n274 = shared-variable-read(w1539, w1529, 100 ("timeout in ms (-1)")) -> (w1538:refnum<k21>, w1509:errorcluster, w1522:T29)  [unwired: 1 out]
        n275 = To Word Integer(number=w1524) -> (16bit integer=w1523:i16)
        n276 = local write "entered"(w1517) -> ()
        n277 = call "helioscan settings to tag settings.vi"("scan specification - helioscan"=w1522) -> ("scan specification - tag resonant"=w1514:T6)  [unwired: 10 in]
        n278 = Bundle By Name(cluster=w1514, "Pockels cell voltage (bits)"=w1523, "lines to delay between scan start and output"="delay scan start", "LSB has acquire control"="LSB has acquire control") -> (w1510:T6)
        n279 = Increment(x=w1528) -> (x+1=w1527:i32)
        "number of update commands received" <- w1527
        n280 = call "setScanPattern.vi"("maximum frequency"="maximum galvo frequency", "error in (no error)"=w1509, "scanning mode"="scanning mode", "Queues"=w1507, "scan specification - tag resonant"=w1510) -> ("error out"=w1508:errorcluster, "scan specification out"=w1502:T6)  [unwired: 5 in]
        n281 = flat-sequence {
          tunnel: [w1543] -> w1531
          tunnel: w1508 -> [w1543]
          frame #0 {
            "scan spec set" <- TRUE ("zIntensity tuples set")
          }
        }
        n282 = xnode "Read/Write Control"("FPGA VI Reference In"=w1504, "scan specification"=w1502) -> ()  [unwired: 1 in, 2 out]
        n283 = local write "scan specification"(w1502) -> ()
        n284 = shared-variable-read(w1537, w1531, 100 ("timeout in ms (-1)"), -1 ("# elements (-1)")) -> (w1536:refnum<k21>, w1513:errorcluster)  [unwired: 2 out]
        n285 = shared-variable-read(w1534, w1513, 100 ("timeout in ms (-1)"), -1 ("# elements (-1)")) -> (w1533:refnum<k21>, w1503:errorcluster)  [unwired: 2 out]
      }
    }
    "finished" <- w1250
    n286 = Unbundle By Name(w1260) -> ("status"=w1259:bool)
    n287 = local read "stop"() -> (w1257:bool)
    n288 = Compound Arithmetic op=OR(w1259, w1261, w1257) -> (w1258:bool)
  }
  n289 = node-c288(w41) -> ()  [unwired: 1 out]
  n290 = local write "stop"(w24) -> ()
  n291 = node-c288(w32) -> ()  [unwired: 1 out]
  n292 = node-c288(w18) -> ()  [unwired: 1 out]
  n293 = local write "stop"(w50) -> ()
  n294 = Merge Errors(w34, w37, w38, w53, w48, w54, w8) -> (w52:errorcluster)
  n295 = flat-sequence {
    tunnel: w52 -> [w1589]
    tunnel: [w1589] -> w71
    frame #0 {
      n296 = local write "stop"(TRUE ("stop")) -> ()
    }
  }
  n297 = flat-sequence {
    tunnel: [w1596] -> w76
    tunnel: w71 -> [w1593]
    tunnel: w51 -> [w1595]
    frame #0 {
      n298 = xnode "Read/Write Control"("FPGA VI Reference In"=w1595, "error in"=w1593, "stop"=TRUE) -> ("FPGA VI Reference Out"=w1594:T13, "error out"=w1592:errorcluster)
      n299 = xnode "Close FPGA VI Reference"("FPGA VI Reference In"=w1594, "error in"=w1592) -> ("error out"=w1596:errorcluster)
    }
  }
  n300 = flat-sequence {
    tunnel: w76 -> [w1643]
    tunnel: [w1643] -> w29
    frame #0 {
      "read loop finished" <- TRUE ("read loop finished")
    }
  }
  n301 = call <vilib>:"Simple Error Handler.vi"("type of dialog (OK msg:1)"=w27, "error in (no error)"=w29) -> ("error out"=w28:errorcluster)  [unwired: 3 in, 4 out]
  n302 = stacked-sequence {
    tunnel: w82 -> [_]
    tunnel: w28 -> [w1644]
    tunnel: [w1644] -> w78
    frame #0 {
      # "reset stop variable"
      n303 = local write "stop"(FALSE) -> ()
    }
  }
  n304 = case "Close front-panel?" shown="True" "Close front-panel?" {
    tunnel: [w1646 w1647] -> _
    tunnel: w78 -> [w1646 w1647]
    frame False {
    }
    frame True {
      n305 = control-ref of="This VI"() -> (w1648:refnum<vi>)
      n306 = invoke class="VI" method="FP.Close"(reference=w1648) -> ()  [unwired: 2 in, 3 out]
    }
  }
  n307 = Destroy Stream Endpoint(11:w83) -> (0:w75:errorcluster)  [unwired: 1 in]
  n308 = flat-sequence {
    tunnel: [w1649] -> w67
    tunnel: w68 -> [w1649]
    frame #0 {
      n309 = local write "stop"(TRUE ("stop")) -> ()
    }
  }
  n310 = Destroy Stream Endpoint(8:w75, 11:w74) -> (0:w73:errorcluster)
  n311 = Destroy Stream Endpoint(8:w73, 11:w72) -> (0:w66:errorcluster)
  n312 = Destroy Stream Endpoint(8:w66, 11:w64) -> (0:w65:errorcluster)
  n313 = Merge Errors(w65, w67, w69) -> (w81:errorcluster)
  n314 = flat-sequence {
    tunnel: w81 -> [w1651]
    tunnel: [w1651] -> w82
    frame #0 {
      n315 = local write "stop"(TRUE ("stop - RT")) -> ()
      "command loop finished" <- TRUE ("command loop finished")
    }
  }
